vi "Pin PPMU configure.vi"(8 "error in (no error)":errorcluster, 10 "Pin config":T1(array[cluster]), 11 "IVI Refnum in":refnum<k15>) -> (0 "error out":errorcluster, 3 "IVI Refnum out":refnum<k15>)   [LabVIEW 2021]
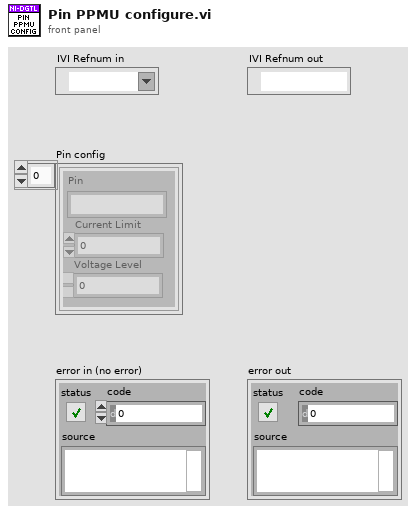
[diagram p1: front panel]
types:
  T1 = cluster{"Pin":string, "Current Limit":dbl, "Voltage Level":dbl}[]
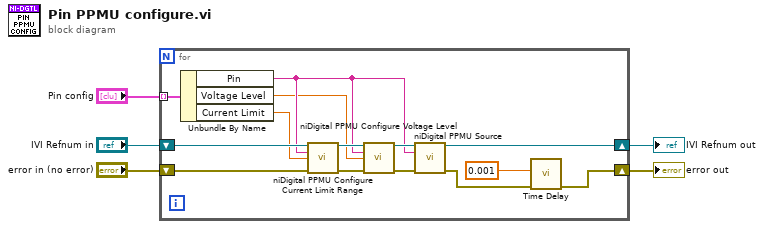
[diagram p0: block diagram]
diagram:
  n1 = for {
    shift-right: [w19] -> w1
    shift-left: "IVI Refnum in" -> [w12]
    shift-right: [w18] -> w2
    shift-left: "error in (no error)" -> [w11]
    tunnel: "Pin config" -> [w10] mode=indexing
    n2 = Unbundle By Name(w10) -> ("Pin"=w8:string, "Voltage Level"=w6:dbl, "Current Limit"=w7:dbl)
    n3 = call <instrlib>:"niDigital PPMU Configure Current Limit Range.vi"("instrument handle"=w12, "channel list"=w8, "current limit range (A)"=w7, "error in"=w11) -> ("instrument handle out"=w16:refnum<k15>, "error out"=w15:errorcluster)  [unwired: 10 in]
    n4 = call <instrlib>:"niDigital PPMU Configure Voltage Level.vi"("instrument handle"=w16, "channel list"=w8, "voltage level (V)"=w6, "error in"=w15) -> ("instrument handle out"=w17:refnum<k15>, "error out"=w14:errorcluster)  [unwired: 10 in]
    n5 = call <instrlib>:"niDigital PPMU Source.vi"("instrument handle"=w17, "channel list"=w8, "error in"=w14) -> ("instrument handle out"=w19:refnum<k15>, "error out"=w13:errorcluster)  [unwired: 11 in]
    n6 = call "Time Delay"("error in (no error)"=w13, "Delay Time (s)"=0.001) -> ("error out"=w18:errorcluster)  [unwired: 9 in]
  }
  "error out" <- w2
  "IVI Refnum out" <- w1
